vi "Read path segments.vi"(8 "error in (no error)":errorcluster, 11 "URI in":refnum<class "URI.lvclass">) -> (0 "error out":errorcluster, 2 "Segments":string[](array[string]), 3 "URI out":refnum<class "URI.lvclass">)   [LabVIEW 2013, in "openURI.lvlib" / "URI.lvclass"]
uses:
  URI.lvclass
  URI.lvclass/URI.ctl
  components/path/URI-Component.Path.lvclass/URI-Component.Path.ctl
  utilities/Percent-Decode String.vi
  components/path/URI-Component.Path.lvclass
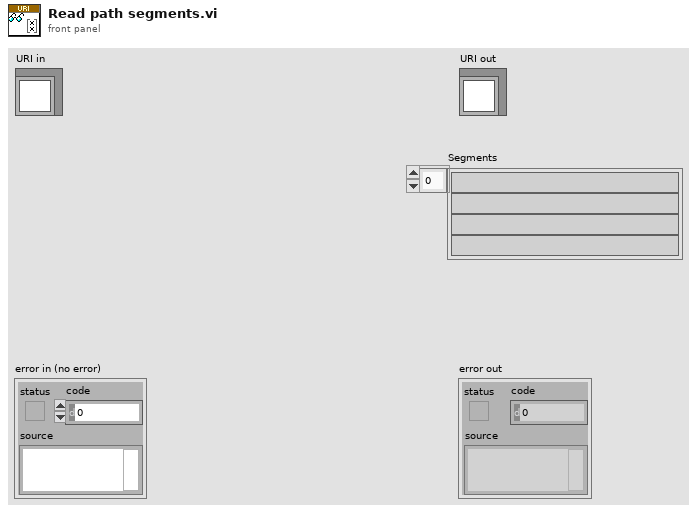
[diagram p1: front panel]
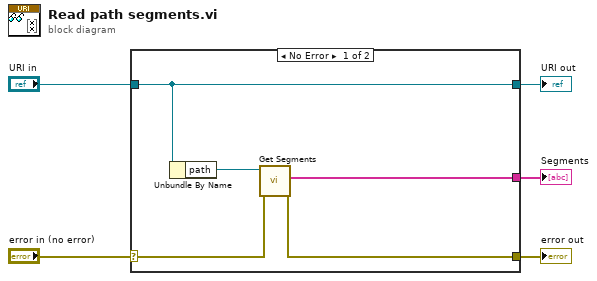
[diagram p0: block diagram]
diagram:
  n1 = case shown="No Error" "error in (no error)" {
    selector: "error in (no error)" -> [w7 w11]
    tunnel: [w6 w11] -> w4
    tunnel: [w10 w12] -> w2
    tunnel: "URI in" -> [w10 w12]
    tunnel: [w8 _] -> w1
    frame No Error {
      n2 = Unbundle By Name(w10) -> ("path"=w9:refnum<class "URI-Component.Path.lvclass">)
      n3 = call "Get Segments.vi"("error in (no error)"=w7, "URI-Component.Path in"=w9) -> ("error out"=w6:errorcluster, "Segments"=w8:string[])  [unwired: 7 in, 1 out]
    }
    frame Error {
    }
  }
  "error out" <- w4
  "URI out" <- w2
  "Segments" <- w1
